vi "update comms status.vi"(6 "comms":enum16{"command", "error", "data"}(ring), 10 "messageHandler in":T1 {"params"."controlChannels"."ballControl" items=["Module6/output0", "Module6/output1", "Module6/output2", "Module6/output3", "Not-Used"]; "params"."controlChannels"."butterflyControl" items=["Module6/output0", "Module6/output1", "Module6/output2", "Module6/output3", "Not-Used"]; "params"."controlChannels"."speedControl" items=["Module6/output0", "Module6/output1", "Module6/output2", "Module6/output3", "Not-Used"]}, 11 "data":variant) -> (0 "this comms":bool, 1 "connection status":bool, 3 "messageHandler out":T1 {"params"."controlChannels"."ballControl" items=["Module6/output0", "Module6/output1", "Module6/output2", "Module6/output3", "Not-Used"]; "params"."controlChannels"."butterflyControl" items=["Module6/output0", "Module6/output1", "Module6/output2", "Module6/output3", "Not-Used"]; "params"."controlChannels"."speedControl" items=["Module6/output0", "Module6/output1", "Module6/output2", "Module6/output3", "Not-Used"]})   [LabVIEW 2018]
uses:
  type defs/message handler data.ctl
  customVI/liveData/state.ctl
panel:
  out "comms status":bool[](array[boolean])
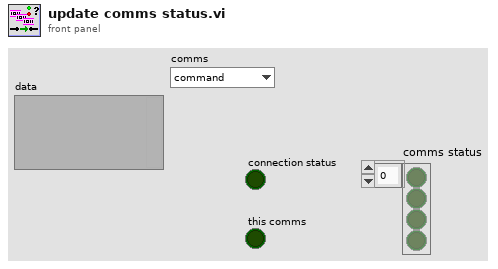
[diagram p1: front panel]
types:
  T1 = typedef "message handler data.ctl" = cluster{"params":cluster{"configFileID":u32, "configFilePath":path, "channelConfigFilePath":path, "incidentLogfile":path, "controlChannels":cluster{"ballControl":u16, "butterflyControl":u16, "speedControl":u16}, "pulsatorVIPath":path, "customVIPath":path, "HowdenAir":cluster{"vent Howden":bool, "Howden%":dbl}}, "vars":cluster{"commsStatus":bool[], "controlIndex":cluster{"ballControl":u16, "butterflyControl":u16, "speedControl":u16}, "customVIRef":refnum<vi>, "Interlocks":cluster{"gearboxOil":bool, "bearingOil":bool, "gearboxAir":bool}, "motorRunning":bool, "liveDataQ":refnum<queue>[]}}
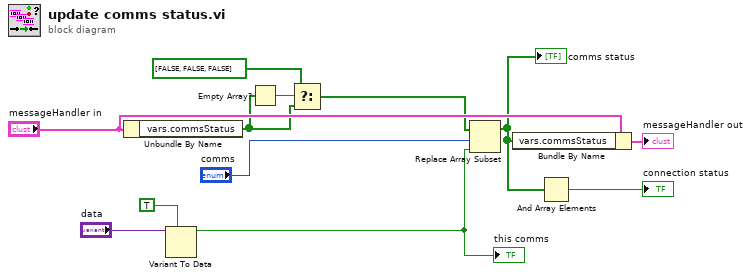
[diagram p0: block diagram]
diagram:
  n1 = Unbundle By Name("messageHandler in") -> ("vars.commsStatus"=w3:bool[])
  n2 = Variant To Data(type=TRUE, Variant="data") -> (data=w7:bool)  [unwired: 1 in, 1 out]
  "this comms" <- w7
  n3 = Empty Array?(array=w3) -> (empty?=w4:bool)
  n4 = Select(t=bool[] [FALSE, FALSE, FALSE], s=w4, f=w3) -> (s? t:f=w1:bool[])
  n5 = Replace Array Subset(array=w1, new element=w7, index="comms") -> (w6:bool[])
  "comms status" <- w6
  n6 = Bundle By Name(cluster="messageHandler in", "vars.commsStatus"=w6) -> (→"messageHandler out":T1)
  n7 = And Array Elements(Boolean array=w6) -> (logical AND=→"connection status":bool)
